vi "Stepper Control3.vi"() -> ()   [LabVIEW 2018]
uses:
  <vilib>/LabVIEW Interface for Arduino/Type Defs/Board Type.ctl
  <vilib>/LabVIEW Interface for Arduino/Type Defs/Connection Type.ctl
  <vilib>/LabVIEW Interface for Arduino/LabVIEW Interface for Arduino.lvlib
panel:
  out "Iteration #":i32
  out "ERROR":errorcluster
  in  "Baud Rate":u32=115200
  out "Step Angle":dbl
  in  "Step Size":i16
  out "Steps Remaining?":bool
  in  "Acceleration":i16
  in  "Set Speed (Steps per Second)":i16=100
  in  "Steps for one rotation":i16
  in  "Control Method":u8(ring)=1 items=["2 Wire (Pulse & Direction)"=1, "2 Wire"=2, "4 Wire"=4, "EasyDriver"=6, "AF Motor Shield (Stepper 1 & 2 Only)"=5]
  in  "Stepper #":u8
  in  "error in":errorcluster
  in  "Board Type (Uno)":T1
  in  "VISA resource":refnum<visa-resource-name>
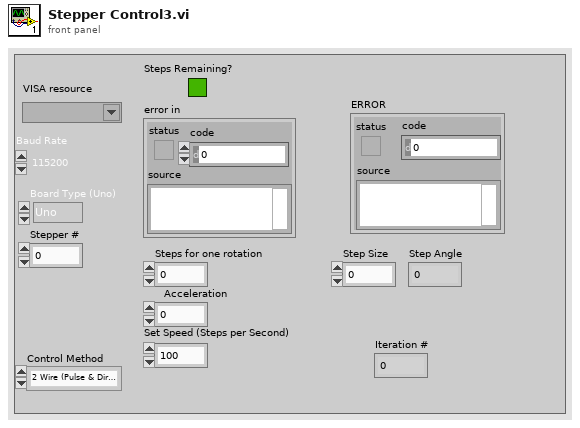
[diagram p1: front panel]
types:
  T1 = typedef "LabVIEW Interface for Arduino.lvlib/Board Type.ctl" = enum16{"Uno", "Dimuelanove w/Atmega 328", "Mega 2560"}
  T2 = typedef "LabVIEW Interface for Arduino.lvlib/Connection Type.ctl" = enum8{"USB / Serial", "XBEE", "BlueSmirf (Bluetooth)"}
  T3 = typedef "LabVIEW Interface for Arduino.lvlib/Arduino Resource.ctl" = cluster{"VISA resource":refnum<visa-resource-name>, "Board Type":T1, "Connection Type":enum8{"USB / Serial"}, "Bytes Per Packet (15)":u8}
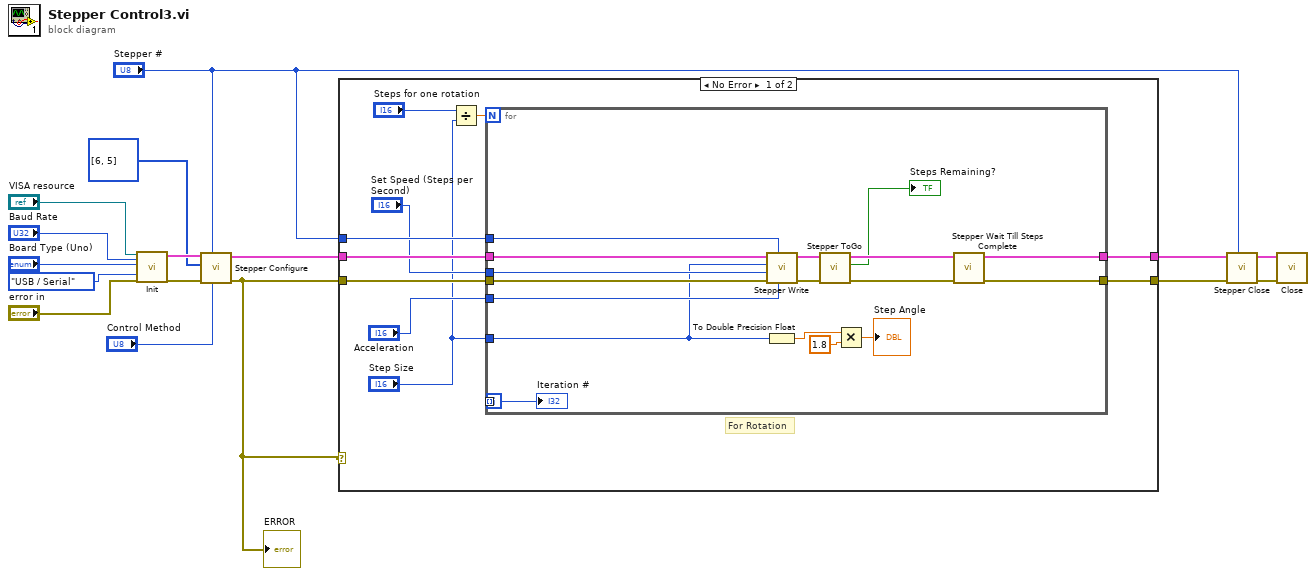
[diagram p0: block diagram]
diagram:
  n1 = call <vilib>:"Init.vi"("VISA resource"="VISA resource", "Baud Rate (115200)"="Baud Rate", "Board Type (Uno)"="Board Type (Uno)", "Connection Type (USB/Serial)"=Connection_Type."USB / Serial", "error in"="error in") -> ("Arduino Resource"=w13:T3, "error out"=w12:errorcluster)  [unwired: 13 in]
  n2 = call <vilib>:"Stepper Configure.vi"("Control Method"="Control Method", "Stepper #"="Stepper #", "error in"=w12, "Stepper Pins"=u8[] [6, 5], "Arduino Resource"=w13) -> ("error out"=w1:errorcluster, "Arduino Resource Out"=w3:T3)  [unwired: 5 in]
  "ERROR" <- w1
  n3 = case shown="No Error" w1 {
    tunnel: [w26 w45] -> w6
    tunnel: [w25 w44] -> w5
    tunnel: "Stepper #" -> [w24 _]
    tunnel: w1 -> [w23 w45]
    tunnel: w3 -> [w22 w44]
    frame No Error {
      # "For Rotation"
      n4 = Divide(x="Steps for one rotation", y="Step Size") -> (x/y=w19:dbl)
      n5 = for {
        N: w19 -> [_]
        tunnel: [w40] -> w26
        tunnel: [w39] -> w25
        tunnel: "Acceleration" -> [w38]
        tunnel: w24 -> [w37]
        tunnel: w23 -> [w36]
        tunnel: "Set Speed (Steps per Second)" -> [w35]
        tunnel: w22 -> [w34]
        tunnel: [w28] -> _ mode=indexing
        tunnel: "Step Size" -> [w27]
        i -> [w28]
        n6 = call <vilib>:"Stepper Write.vi"("Set Acceleration (0 to disable)"=w38, "Stepper #"=w37, "error in"=w36, "Set Speed (Steps per Second)"=w35, "# of Steps to Move"=w27, "Arduino Resource"=w34) -> ("error out"=w33:errorcluster, "Arduino Resource Out"=w32:T3)  [unwired: 4 in]
        n7 = To Double Precision Float(number=w27) -> (double precision float=w30:dbl)
        n8 = call <vilib>:"Stepper ToGo.vi"("error in"=w33, "Arduino Resource"=w32) -> ("error out"=w43:errorcluster, "Steps Remaining?"=→"Steps Remaining?":bool, "Arduino Resource Out"=w42:T3)  [unwired: 6 in, 1 out]
        n9 = Multiply(x=w30, y=1.8) -> (x*y=→"Step Angle":dbl)
        n10 = call <vilib>:"Stepper Wait Till Steps Complete.vi"("error in"=w43, "Arduino Resource In"=w42) -> ("error out"=w40:errorcluster, "Arduino Resource Out"=w39:T3)  [unwired: 8 in]
        "Iteration #" <- w28
      }
    }
    frame Error {
    }
  }
  n11 = call <vilib>:"Stepper Close.vi"("Stepper #"="Stepper #", "error in"=w6, "Arduino Resource"=w5) -> ("error out"=w7:errorcluster, "Arduino Resource Out"=w8:T3)  [unwired: 7 in]
  n12 = call <vilib>:"Close.vi"("Arduino Resource"=w8, "error in"=w7) -> ()  [unwired: 13 in, 1 out]
